vi "Harvest_Folder_Client.vi"(4 "Age in Days of files":dbl=nan, 5 "Get all Server Files":bool, 6 "Check Updates on Server?":bool, 7 "Archive Files?":bool, 8 "Folder to Harvest":path=path "/Lacie_20/EnFlo_Data/Andrew_Burt/Results") -> (0 "error out":errorcluster, 1 "Files to Pull From Server":path[](array[path]), 2 "Files to Push to Server":path[](array[path]), 3 "Folder contents changed?":bool)   [LabVIEW 2015]
uses:
  Sub VIs/Harvest_Global.vi
  Anemometry/Anemometry Sub Vis/Globals/Preference_global.vi
  Anemometry/Anemometry Sub Vis/Globals/Constants_global.vi
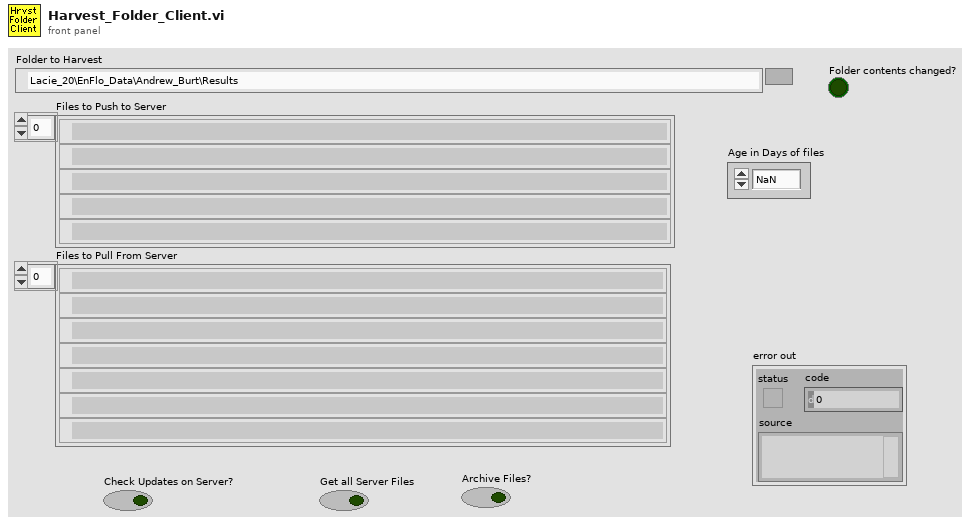
[diagram p1: front panel]
types:
  T1 = typedef "Server_Comms.ctl" = enum16{"Server Link Healthy", "Do Not Link To Server"}
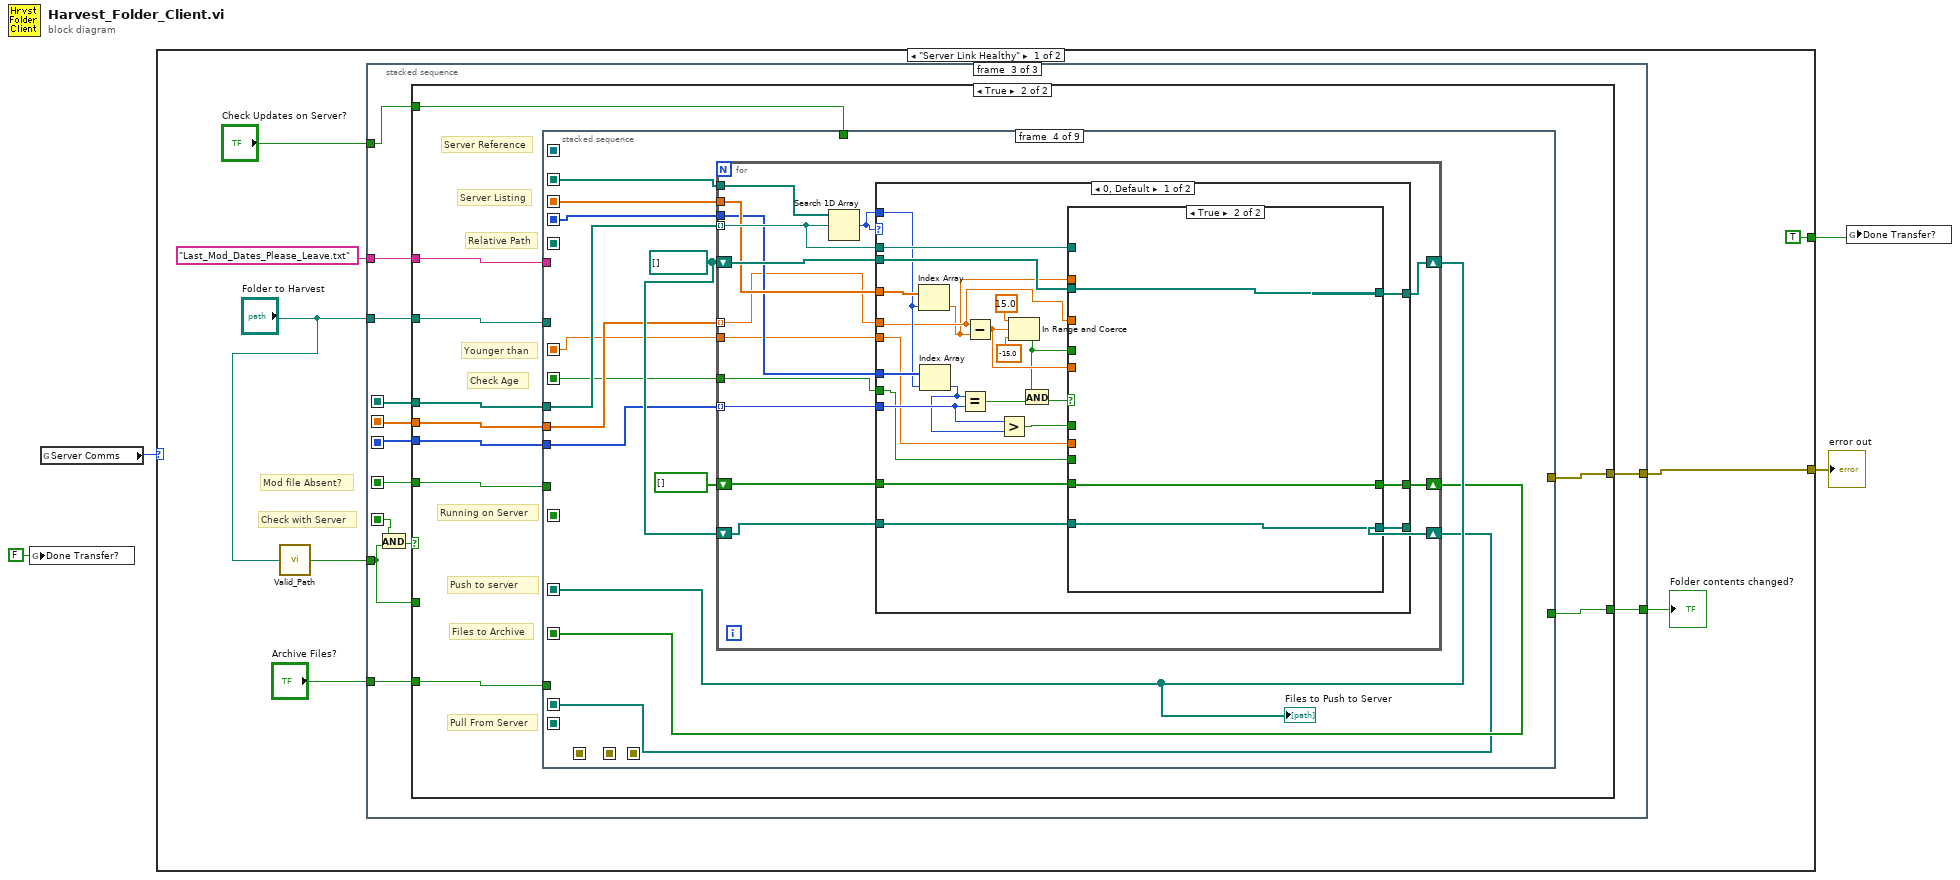
[diagram p0: block diagram]
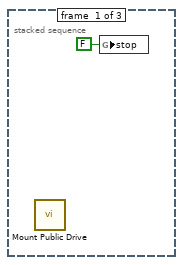
[diagram p2: hidden frame]
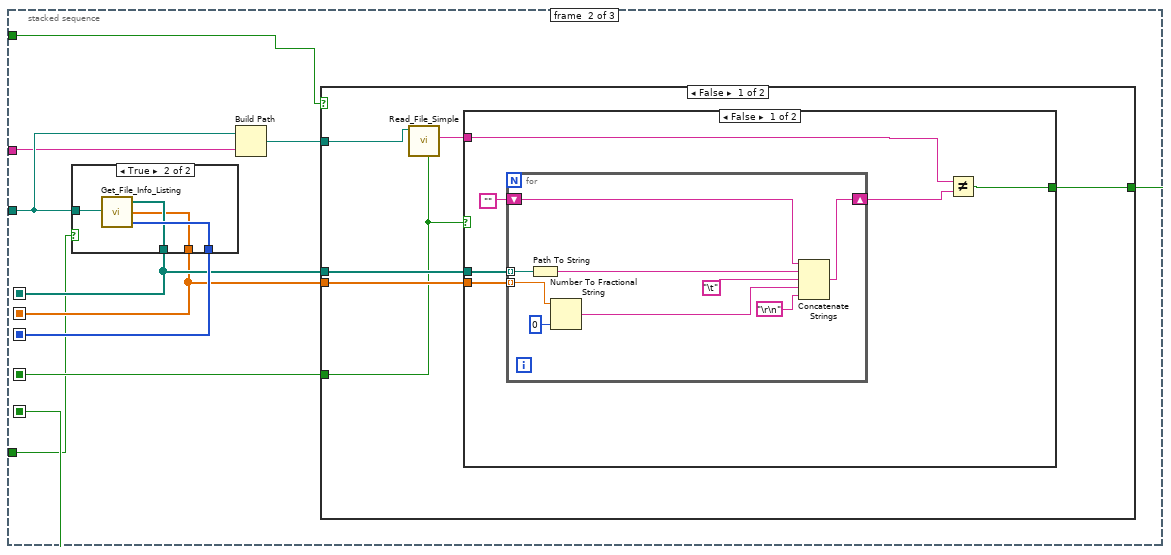
[diagram p3: hidden frame]
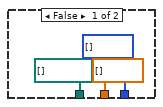
[diagram p4: hidden frame]
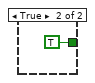
[diagram p5: hidden frame]
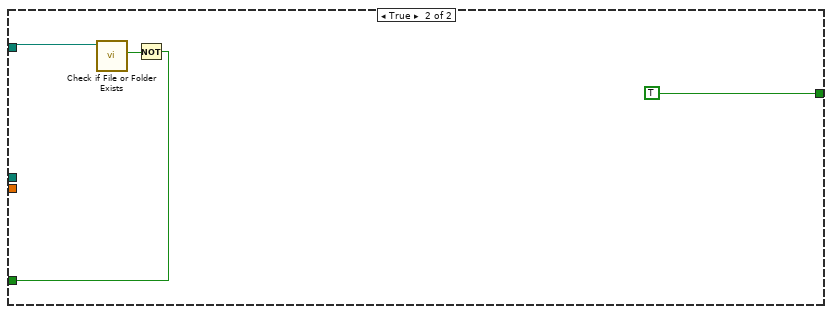
[diagram p6: hidden frame]
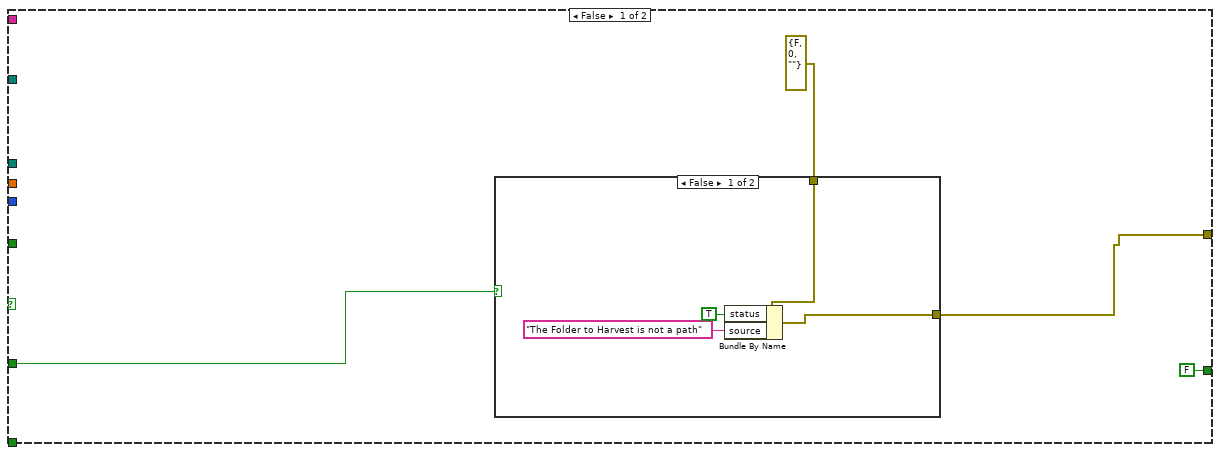
[diagram p7: hidden frame]
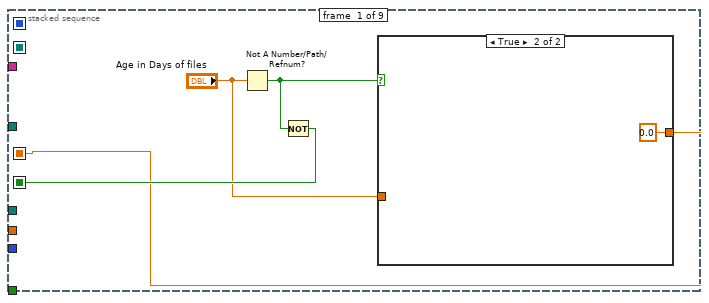
[diagram p9: hidden frame]
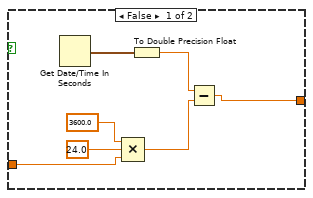
[diagram p10: hidden frame]
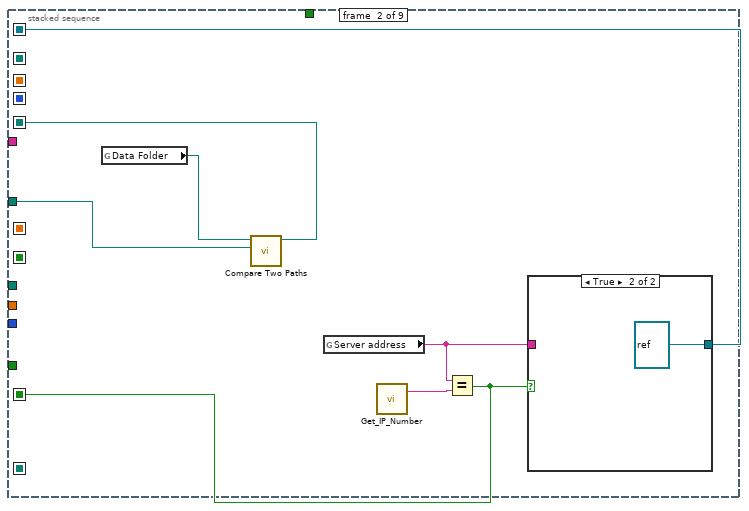
[diagram p11: hidden frame]
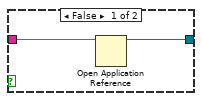
[diagram p12: hidden frame]
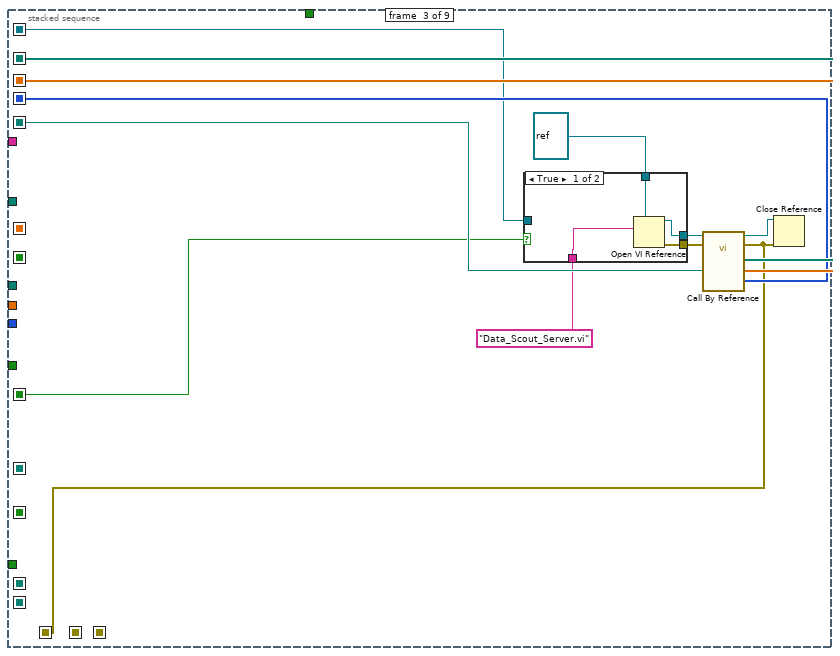
[diagram p13: hidden frame]
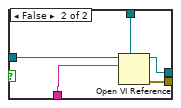
[diagram p14: hidden frame]
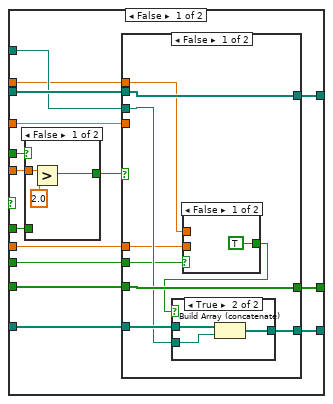
[diagram p15: hidden frame]
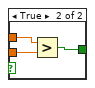
[diagram p18: hidden frame]
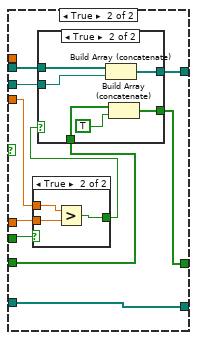
[diagram p19: hidden frame]
diagram:
  n1 = global write "Harvest_Global.vi" "Done Transfer?"(FALSE ("Done Transfer?")) -> ()
  n2 = global read "Preference_global.vi" "Server Comms"() -> (w4:T1)
  n3 = case shown="\"Server Link Healthy\"" w4 {
    tunnel: [w6 w366] -> w3
    tunnel: [TRUE ("Done Transfer?") TRUE ("Done Transfer?")] -> w1
    frame "Server Link Healthy" {
      # "Mod file Absent?"
      # "Check with Server"
      n4 = call "Valid_Path.vi"("Filename"="Folder to Harvest") -> ("Valid Path?"=w9:bool)
      n5 = stacked-sequence {
        seq-local: [_ w22 _] -> [_ _ w68]
        seq-local: [_ w21 _] -> [_ _ w67]
        seq-local: [_ w23 _] -> [_ _ w66]
        seq-local: [_ w20 _] -> [_ _ w61]
        seq-local: [_ w19 _] -> [_ _ w62]
        tunnel: "Folder to Harvest" -> [_ w18 w69]
        tunnel: "Last_Mod_Dates_Please_Leave.txt" ("name or relative path") -> [_ w17 w65]
        tunnel: [_ _ w64] -> w6
        tunnel: [_ _ w63] -> w11
        tunnel: w9 -> [_ w15 w59]
        tunnel: "Archive Files?" -> [_ _ w58]
        tunnel: "Check Updates on Server?" -> [_ w14 w57]
        frame #0 {
          n6 = call "Mount Public Drive.vi"() -> ()  [unwired: 12 in]
          n7 = global write "Harvest_Global.vi" "stop"(FALSE ("stop")) -> ()
        }
        frame #1 {
          n8 = case shown="True" w15 {
            tunnel: [i64[] [] ("Size") w30] -> w23
            tunnel: [path[] [] ("Path") w29] -> w22
            tunnel: [dbl[] [] ("Last Mod") w28] -> w21
            tunnel: w18 -> [_ w27]
            frame False {
            }
            frame True {
              n9 = call "Get_File_Info_Listing.vi"("path"=w27) -> ("Path"=w29:path[], "Last Mod"=w28:dbl[], "Size"=w30:i64[])
            }
          }
          n10 = Build Path(base path=w18, name or relative path=w17) -> (appended path=w16:path)
          n11 = case shown="False" w14 {
            tunnel: w22 -> [w36 _]
            tunnel: w21 -> [w35 _]
            tunnel: [w33 TRUE] -> w20
            tunnel: [w32 w53] -> w19
            tunnel: w16 -> [w31 w55]
            frame False {
              n12 = call "Read_File_Simple.vi"("Filename"=w31) -> ("Error?"=w32:bool, "string"=w34:string)  [unwired: 4 in, 4 out]
              n13 = case shown="False" w32 {
                tunnel: w36 -> [w41 _]
                tunnel: w35 -> [w40 _]
                tunnel: w34 -> [w39 _]
                tunnel: [w37 TRUE] -> w33
                frame False {
                  n14 = for {
                    tunnel: w41 -> [w51] mode=indexing
                    tunnel: w40 -> [w49] mode=indexing
                    shift-right: [w43] -> w38
                    shift-left: "" -> [w48]
                    n15 = Path To String(path=w51) -> (string=w47:string)
                    n16 = Number To Fractional String(number=w49, precision (6)=i16 0) -> (F-format string=w45:string)  [unwired: 2 in]
                    n17 = Concatenate Strings(w48, w47, "\t", w45, "\r\n") -> (w43:string)
                  }
                  n18 = Not Equal?(x=w39, y=w38) -> (x != y?=w37:bool)
                }
                frame True {
                }
              }
            }
            frame True {
              n19 = call <vilib>:"Check if File or Folder Exists.vi"("path"=w55) -> ("file or folder exists?"=w54:bool)  [unwired: 8 in, 2 out]
              n20 = Not(x=w54) -> (.not. x?=w53:bool)
            }
          }
        }
        frame #2 {
          n21 = And(x=w61, y=w59) -> (x .and. y?=w60:bool)
          n22 = case shown="True" w60 {
            tunnel: w69 -> [_ w88]
            tunnel: w68 -> [_ w87]
            tunnel: w67 -> [_ w86]
            tunnel: w66 -> [_ w85]
            tunnel: w65 -> [_ w84]
            tunnel: [w70 w83] -> w64
            tunnel: [FALSE w82] -> w63
            tunnel: w62 -> [_ w81]
            tunnel: w59 -> [w72 _]
            tunnel: w58 -> [_ w80]
            tunnel: w57 -> [_ w79]
            frame False {
              n23 = case shown="False" w72 {
                tunnel: errorcluster {"status"=FALSE, "code"=0, "source"=""} ("Error IO") -> [w77 w78]
                tunnel: [w74 w78] -> w70
                frame False {
                  n24 = Bundle By Name(cluster=w77, "status"=TRUE, "source"="The Folder to Harvest is not a path") -> (w74:errorcluster)
                }
                frame True {
                }
              }
            }
            frame True {
              # "Younger than"
              # "Check Age"
              # "Running on Server"
              # "Server Reference"
              # "Pull From Server"
              # "Server Listing"
              # "Relative Path"
              # "Files to Archive"
              # "Push to server"
              n25 = stacked-sequence {
                seq-local: [_ _ w119 _ _ _ _ _ _] -> [_ _ _ w144 _ w287 _ _ _]
                seq-local: [_ _ w118 _ _ _ _ _ _] -> [_ _ _ w143 _ w280 _ _ _]
                seq-local: [_ _ _ w142 _ _ _ _ _] -> [_ _ _ _ w268 _ _ w341 _]
                seq-local: [_ _ _ w141 _ _ _ _ _] -> [_ _ _ _ w273 _ _ _ _]
                seq-local: [_ w105 _ _ _ _ _ _ _] -> [_ _ w120 _ w270 _ w327 _ _]
                seq-local: [_ _ w117 _ _ _ _ _ _] -> [_ _ _ w138 _ _ _ _ _]
                seq-local: [_ _ _ w137 _ _ _ _ _] -> [_ _ _ _ _ w286 _ _ _]
                seq-local: [_ w104 _ _ _ _ _ _ _] -> [_ _ w112 _ w275 _ w326 _ w361]
                seq-local: [_ _ w113 _ _ _ _ _ _] -> [_ _ _ _ w269 _ _ _ _]
                seq-local: [_ _ _ _ w274 _ _ _ _] -> [_ _ _ _ _ _ w323 _ _]
                seq-local: [_ _ _ _ _ w285 _ _ _] -> [_ _ _ _ _ _ w321 w340 _]
                seq-local: [_ _ _ _ _ _ w322 _ _] -> [_ _ _ _ _ _ _ w334 _]
                seq-local: [_ w101 _ _ _ _ _ _ _] -> [_ _ w111 _ w276 _ w325 _ w362]
                seq-local: [w91 _ _ _ _ _ _ _ _] -> [_ _ _ w133 _ w282 _ _ _]
                seq-local: [w90 _ _ _ _ _ _ _ _] -> [_ _ _ w132 _ w281 _ _ _]
                tunnel: w88 -> [_ w106 _ _ _ _ _ w336 _]
                tunnel: w87 -> [_ _ _ w136 _ w284 _ _ _]
                tunnel: w86 -> [_ _ _ w135 _ _ _ _ _]
                tunnel: w85 -> [_ _ _ w134 _ _ _ _ _]
                tunnel: w84 -> [_ _ _ _ _ _ _ w335 _]
                tunnel: [_ _ _ _ _ _ _ w334 _] -> w83
                tunnel: [_ _ _ _ _ _ _ w333 _] -> w82
                tunnel: w81 -> [_ _ _ _ _ _ _ w332 _]
                tunnel: w80 -> [_ _ _ _ w272 _ w324 _ _]
                tunnel: w79 -> [_ _ _ _ _ w283 _ _ _]
                frame #0 {
                  n26 = Not A Number/Path/Refnum?(number/path/refnum="Age in Days of files") -> (NaN/Path/Refnum?=w92:bool)
                  n27 = Not(x=w92) -> (.not. x?=w91:bool)
                  n28 = case shown="True" w92 {
                    tunnel: [w93 0.0] -> w90
                    tunnel: "Age in Days of files" -> [w95 _]
                    frame False {
                      n29 = Get Date/Time In Seconds() -> (seconds since 1Jan1904=w99:timestamp)
                      n30 = Compound Arithmetic op=MULTIPLY(3600.0, 24.0, w95) -> (w94:dbl)
                      n31 = To Double Precision Float(number=w99) -> (double precision float=w98:dbl)
                      n32 = Subtract(x=w98, y=w94) -> (x-y=w93:dbl)
                    }
                    frame True {
                    }
                  }
                }
                frame #1 {
                  n33 = global read "Constants_global.vi" "Data Folder"() -> (w107:path)
                  n34 = call <vilib>:"Compare Two Paths.vi"("Path 2"=w106, "Path 1"=w107) -> ("Relative Path from 1 to 2"=w105:path)  [unwired: 6 in, 3 out]
                  n35 = global read "Preference_global.vi" "Server address"() -> (w103:string)
                  n36 = call "Get_IP_Number.vi"() -> ("IP Number"=w102:string)  [unwired: 1 out]
                  n37 = Equal?(x=w103, y=w102) -> (x = y?=w101:bool)
                  n38 = case shown="True" w101 {
                    tunnel: [w109 refnum<vi> refnum ("application reference (local)")] -> w104
                    tunnel: w103 -> [w108 _]
                    frame False {
                      n39 = Open Application Reference(11:w108) -> (3:w109:refnum<vi>)  [unwired: 2 in, 2 out]
                    }
                    frame True {
                    }
                  }
                }
                frame #2 {
                  n40 = case shown="True" w111 {
                    tunnel: [w126 w131] -> w122
                    tunnel: [w125 w130] -> w121
                    tunnel: "Data_Scout_Server.vi" -> [w124 w129]
                    tunnel: refnum<vi> refnum ("Scout Server") -> [w123 w128]
                    tunnel: w112 -> [_ w127]
                    frame True {
                      n41 = Open VI Reference(type specifier VI Refnum (for type only)=w123, vi path=w124) -> (vi reference=w126:refnum<vi>, error out=w125:errorcluster)  [unwired: 2 in, 2 out]
                    }
                    frame False {
                      n42 = Open VI Reference(type specifier VI Refnum (for type only)=w128, application reference (local)=w127, vi path=w129) -> (vi reference=w131:refnum<vi>, error out=w130:errorcluster)  [unwired: 1 in, 2 out]
                    }
                  }
                  n43 = call-by-ref "?"(reference=w122, error in=w121, "Relative Path"=w120) -> (reference out=w116:refnum<vi>, error out=w113:errorcluster, "Path"=w119:path[], "Last Mod"=w118:dbl[], "Size"=w117:i64[])
                  n44 = Close Reference(reference=w116, error in (no error)=w113) -> ()  [unwired: 1 out]
                }
                frame #3 {
                  w139 = path[] []
                  n45 = for {
                    tunnel: w136 -> [w158] mode=indexing
                    shift-right: [w148] -> w142
                    shift-left: w139 -> [w159]
                    tunnel: w144 -> [w157]
                    tunnel: w143 -> [w155]
                    tunnel: w135 -> [w147] mode=indexing
                    shift-right: [w153] -> w141
                    shift-left: bool[] [] -> [w154]
                    shift-right: [w151] -> w137
                    shift-left: w139 -> [w152]
                    tunnel: w138 -> [w150]
                    tunnel: w134 -> [w149] mode=indexing
                    tunnel: w133 -> [w146]
                    tunnel: w132 -> [w145]
                    n46 = Search 1D Array(1D array=w157, element=w158) -> (index of element=w156:i32)  [unwired: 1 in]
                    n47 = case shown="0, Default" w156 {
                      tunnel: w159 -> [w180 w253]
                      tunnel: [w181 w252] -> w148
                      tunnel: w158 -> [w179 w251]
                      tunnel: w156 -> [w170 _]
                      tunnel: w155 -> [w182 _]
                      tunnel: w147 -> [w161 w245]
                      tunnel: w154 -> [w175 w250]
                      tunnel: [w174 w249] -> w153
                      tunnel: w152 -> [w173 w248]
                      tunnel: [w172 w248] -> w151
                      tunnel: w150 -> [w171 _]
                      tunnel: w149 -> [w169 _]
                      tunnel: w146 -> [w163 w247]
                      tunnel: w145 -> [w162 w244]
                      frame 0, Default {
                        n48 = Index Array(array=w182, index=w170) -> (element=w160:dbl)
                        n49 = Index Array(array=w171, index=w170) -> (element=w168:i64)
                        n50 = Equal?(x=w168, y=w169) -> (x = y?=w167:bool)
                        n51 = Subtract(x=w161, y=w160) -> (x-y=w176:dbl)
                        n52 = Greater?(x=w169, y=w168) -> (0:w166:bool)
                        n53 = In Range and Coerce(upper limit=15.0, x=w176, lower limit=-15.0) -> (In Range?=w165:bool)  [unwired: 1 out]
                        n54 = And(x=w165, y=w167) -> (x .and. y?=w164:bool)
                        n55 = case shown="True" w164 {
                          tunnel: [w197 w243] -> w181
                          tunnel: w180 -> [w196 w243]
                          tunnel: w179 -> [w195 _]
                          tunnel: w176 -> [w194 _]
                          tunnel: w175 -> [w193 w242]
                          tunnel: [w192 w242] -> w174
                          tunnel: w173 -> [w191 w241]
                          tunnel: [w190 w241] -> w172
                          tunnel: w166 -> [w189 _]
                          tunnel: w165 -> [w188 _]
                          tunnel: w163 -> [w186 _]
                          tunnel: w162 -> [w185 _]
                          tunnel: w161 -> [w184 _]
                          tunnel: w160 -> [w183 _]
                          frame False {
                            n56 = case shown="False" w188 {
                              tunnel: [w200 w201] -> w187
                              tunnel: w194 -> [w199 _]
                              tunnel: w189 -> [_ w201]
                              frame False {
                                n57 = Greater?(x=w199, y=2.0) -> (0:w200:bool)
                              }
                              frame True {
                              }
                            }
                            n58 = case shown="False" w187 {
                              tunnel: [w210 w228] -> w197
                              tunnel: w196 -> [w210 w227]
                              tunnel: w195 -> [w206 w226]
                              tunnel: w193 -> [w209 w222]
                              tunnel: [w209 w223] -> w192
                              tunnel: w191 -> [w208 w225]
                              tunnel: [w207 w225] -> w190
                              tunnel: w186 -> [w205 w221]
                              tunnel: w185 -> [w204 w220]
                              tunnel: w184 -> [_ w219]
                              tunnel: w183 -> [w202 _]
                              frame False {
                                n59 = case shown="False" w205 {
                                tunnel: w202 -> [_ w218]
                                tunnel: w204 -> [_ w217]
                                tunnel: [TRUE w216] -> w203
                                frame False {
                                }
                                frame True {
                                n60 = Greater?(x=w218, y=w217) -> (0:w216:bool)
                                }
                                }
                                n61 = case shown="True" w203 {
                                tunnel: w208 -> [w211 w214]
                                tunnel: [w211 w213] -> w207
                                tunnel: w206 -> [_ w212]
                                frame False {
                                }
                                frame True {
                                n62 = Build Array (concatenate)(w214, w212) -> (w213:path[])
                                }
                                }
                              }
                              frame True {
                                n63 = case shown="True" w221 {
                                tunnel: w219 -> [_ w240]
                                tunnel: w220 -> [_ w239]
                                tunnel: [TRUE w238] -> w224
                                frame False {
                                }
                                frame True {
                                n64 = Greater?(x=w240, y=w239) -> (0:w238:bool)
                                }
                                }
                                n65 = case shown="True" w224 {
                                tunnel: [w229 w236] -> w228
                                tunnel: w227 -> [w229 w235]
                                tunnel: w226 -> [_ w234]
                                tunnel: [w230 w232] -> w223
                                tunnel: w222 -> [w230 w231]
                                frame False {
                                }
                                frame True {
                                n66 = Build Array (concatenate)(w235, w234) -> (w236:path[])
                                n67 = Build Array (concatenate)(w231, TRUE) -> (w232:bool[])
                                }
                                }
                              }
                            }
                          }
                          frame True {
                          }
                        }
                      }
                      frame -1 {
                        n68 = case shown="True" w247 {
                          tunnel: w245 -> [_ w257]
                          tunnel: w244 -> [_ w256]
                          tunnel: [TRUE w255] -> w246
                          frame False {
                          }
                          frame True {
                            n69 = Greater?(x=w257, y=w256) -> (0:w255:bool)
                          }
                        }
                        n70 = case shown="True" w246 {
                          tunnel: w253 -> [w259 w265]
                          tunnel: [w259 w264] -> w252
                          tunnel: w251 -> [_ w263]
                          tunnel: w250 -> [w258 w262]
                          tunnel: [w258 w261] -> w249
                          frame False {
                          }
                          frame True {
                            n71 = Build Array (concatenate)(w262, FALSE) -> (w261:bool[])
                            n72 = Build Array (concatenate)(w265, w263) -> (w264:path[])
                          }
                        }
                      }
                    }
                  }
                  "Files to Push to Server" <- w142
                }
                frame #4 {
                  n73 = Array Size(array=w268) -> (size(s)=w267:i32)
                  n74 = global write "Harvest_Global.vi" "No Files to Push"(w267) -> ()
                  n75 = And(x=w273, y=w272) -> (x .and. y?=w271:bool[])
                  n76 = for {
                    tunnel: w270 -> [w279]
                    tunnel: w268 -> [w278] mode=indexing
                    tunnel: [w277] -> w266 mode=indexing
                    n77 = Build Path(base path=w279, name or relative path=w278) -> (appended path=w277:path)
                  }
                  n78 = call "Push_Data_via_Public_Client.vi"("Archive File?"=w271, "application reference"=w275, "error in (no error)"=w269, "Running on Server?"=w276, "Path of Files relative to EnFlo Data Root"=w266) -> ("error out"=w274:errorcluster)  [unwired: 5 in]
                }
                frame #5 {
                  n79 = case shown="True" "Get all Server Files" {
                    tunnel: w284 -> [_ w299]
                    tunnel: w287 -> [_ w298]
                    tunnel: w286 -> [w291 w297]
                    tunnel: [w290 w296] -> w285
                    tunnel: w283 -> [w292 _]
                    tunnel: w282 -> [_ w295]
                    tunnel: w281 -> [_ w294]
                    tunnel: w280 -> [_ w293]
                    frame False {
                      n80 = Select(t=w291, s=w292, f=path[] []) -> (s? t:f=w290:path[])
                    }
                    frame True {
                      n81 = for {
                        tunnel: w298 -> [w309] mode=indexing
                        shift-right: [w307] -> w296
                        shift-left: w297 -> [w310]
                        tunnel: w299 -> [w308]
                        tunnel: w295 -> [w306]
                        tunnel: w294 -> [w305]
                        tunnel: w293 -> [w304] mode=indexing
                        n82 = case shown="True" w306 {
                          tunnel: w304 -> [_ w314]
                          tunnel: w305 -> [_ w313]
                          tunnel: [TRUE w312] -> w300
                          frame False {
                          }
                          frame True {
                            n83 = Greater?(x=w314, y=w313) -> (0:w312:bool)
                          }
                        }
                        n84 = Search 1D Array(1D array=w308, element=w309) -> (index of element=w303:i32)  [unwired: 1 in]
                        n85 = Less Than 0?(x=w303) -> (x < 0?=w301:bool)
                        n86 = And(x=w301, y=w300) -> (x .and. y?=w302:bool)
                        n87 = case shown="True" w302 {
                          tunnel: w310 -> [w315 w318]
                          tunnel: [w315 w317] -> w307
                          tunnel: w309 -> [_ w316]
                          frame False {
                          }
                          frame True {
                            n88 = Build Array (concatenate)(w318, w316) -> (w317:path[])
                          }
                        }
                      }
                    }
                  }
                }
                frame #6 {
                  n89 = Array Size(array=w321) -> (size(s)=w320:i32)
                  n90 = for {
                    tunnel: w327 -> [w330]
                    tunnel: w321 -> [w329] mode=indexing
                    tunnel: [w328] -> w319 mode=indexing
                    n91 = Build Path(base path=w330, name or relative path=w329) -> (appended path=w328:path)
                  }
                  n92 = global write "Harvest_Global.vi" "No Files to Pull"(w320) -> ()
                  n93 = call "Pull_Data_via_Public_Client.vi"("application reference"=w326, "error in (no error)"=w323, "Archive Files?"=w324, "Running on Server?"=w325, "Path of File relative to EnFlo Data Root"=w319) -> ("error out"=w322:errorcluster)  [unwired: 1 in]
                  "Files to Pull From Server" <- w321
                }
                frame #7 {
                  n94 = Array Size(array=w340) -> (size(s)=w338:i32)
                  n95 = Array Size(array=w341) -> (size(s)=w339:i32)
                  n96 = Add(x=w339, y=w338) -> (x+y=w337:i32)
                  n97 = Greater Than 0?(x=w337) -> (x > 0?=w333:bool)
                  n98 = Or(x=w332, y=w333) -> (x .or. y?=w331:bool)
                  n99 = case shown="No Error" w334 {
                    tunnel: w336 -> [w344 _]
                    tunnel: w335 -> [w343 _]
                    tunnel: w331 -> [w342 _]
                    frame No Error {
                      n100 = case shown="True" w342 {
                        tunnel: w344 -> [_ w347]
                        tunnel: w343 -> [_ w345]
                        frame False {
                        }
                        frame True {
                          n101 = call "Get_File_Info_Listing.vi"("path"=w347) -> ("Path"=w351:path[], "Last Mod"=w350:dbl[])  [unwired: 1 out]
                          n102 = for {
                            tunnel: w351 -> [w360] mode=indexing
                            tunnel: w350 -> [w358] mode=indexing
                            shift-right: [w352] -> w348
                            shift-left: "" -> [w357]
                            n103 = Path To String(path=w360) -> (string=w356:string)
                            n104 = Number To Fractional String(number=w358, precision (6)=i16 0) -> (F-format string=w354:string)  [unwired: 2 in]
                            n105 = Concatenate Strings(w357, w356, "\t", w354, "\r\n") -> (w352:string)
                          }
                          n106 = Build Path(base path=w347, name or relative path=w345) -> (appended path=w346:path)
                          n107 = call "Write_File_Simple.vi"("character string"=w348, "file path"=w346) -> ()  [unwired: 1 in, 2 out]
                        }
                      }
                    }
                    frame Error {
                    }
                  }
                }
                frame #8 {
                  n108 = case shown="False" w362 {
                    tunnel: w361 -> [w363 _]
                    frame False {
                      n109 = Close Reference(reference=w363) -> ()  [unwired: 1 in, 1 out]
                    }
                    frame True {
                    }
                  }
                }
              }
            }
          }
        }
      }
      "Folder contents changed?" <- w11
    }
    frame "Do Not Link To Server" {
      n110 = Bundle By Name(cluster=errorcluster {"status"=FALSE, "code"=0, "source"=""} ("Error IO"), "status"=TRUE, "source"="Preference Panel set to \"Do Not Link To Server\"") -> (w366:errorcluster)
    }
  }
  "error out" <- w3
  n111 = global write "Harvest_Global.vi" "Done Transfer?"(w1) -> ()
